vi "FGV Parameters.vi"(7 "CMD":T1, 8 "error in (no error)":errorcluster, 10 "input":variant, 11 "Key":string) -> (0 "error out":errorcluster, 2 "output":variant, 3 "FVG Variant":variant)   [LabVIEW 2020]
uses:
  PCT FGV CMD.ctl
panel:
  # "0 - Gage at Zero\n1 - GF"
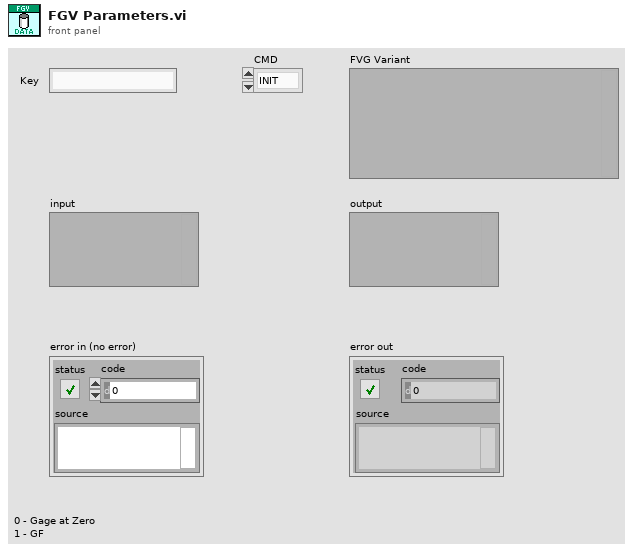
[diagram p1: front panel]
types:
  T1 = typedef "PCT FGV CMD.ctl" = enum16{"INIT", "GET", "SET"}
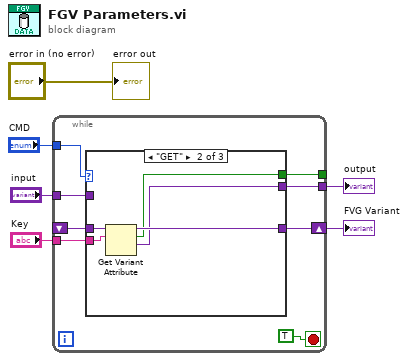
[diagram p0: block diagram]
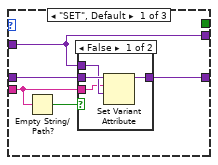
[diagram p2: hidden frame]
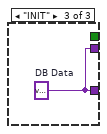
[diagram p4: hidden frame]
diagram:
  n1 = while {
    tunnel: "input" -> [w12]
    tunnel: "CMD" -> [w14]
    shift-right: [w11] -> w6
    shift-left: _ -> [w13]
    tunnel: "Key" -> [w9]
    tunnel: [w8] -> w5
    tunnel: [w7] -> _
    stop <- TRUE stop-if-true
    n2 = case shown="\"GET\"" w14 {
      tunnel: w13 -> [w19 w29 _]
      tunnel: w12 -> [w17 _ _]
      tunnel: [w18 w27 w30] -> w11
      tunnel: w9 -> [w16 w28 _]
      tunnel: [w17 w26 w30] -> w8
      tunnel: [_ w25 _] -> w7
      frame "SET", Default {
        n3 = Empty String/Path?(string/path=w16) -> (empty?=w15:bool)
        n4 = case shown="False" w15 {
          tunnel: w19 -> [w23 w24]
          tunnel: [w22 w24] -> w18
          tunnel: w17 -> [w21 _]
          tunnel: w16 -> [w20 _]
          frame False {
            n5 = Set Variant Attribute(Variant=w23, name=w20, value=w21) -> (Variant out=w22:variant)  [unwired: 1 in, 2 out]
          }
          frame True {
          }
        }
      }
      frame "GET" {
        n6 = Get Variant Attribute(Variant=w29, name=w28) -> (duplicate Variant=w27:variant, found=w25:bool, value=w26:variant)  [unwired: 2 in, 1 out]
      }
      frame "INIT" {
        w30 = variant  # DB Data
      }
    }
  }
  "FVG Variant" <- w6
  "output" <- w5
  "error out" <- "error in (no error)"
